vi "Handle Time Domain Data.vi"(8 "error in":errorcluster, 10 "Spkeaker On?":bool=TRUE, 11 "Cell Data in":refnum<class "PAS Cell Data.lvclass">) -> (0 "error out":errorcluster, 3 "Cell Data out":refnum<class "PAS Cell Data.lvclass">)   [LabVIEW 2014, in "PAS Library.lvlib" / "PAS Cell Data.lvclass"]
doc: "This VI handles the time domain data and any necessary transformation into the frequency domain. If the speaker is on, then the frequency domain data for the mic returned is the power spectrum (magnitude squared) and if the speaker is off, then the desired result is the magnitude. \n\nAlso, if the speaker is off, then the phase at the resonant frequency for the mic and photodiode are stored."
uses:
  PAS Cell Data.lvclass
  <vilib>/Analysis/4window.llb/windowTd.ctl
  PAS Cell Data.lvclass/PAS Cell Data.ctl
  <vilib>/measure/maspectr.llb/FFT Spectrum (Mag-Phase) for 1 Chan.vi
  <vilib>/Analysis/NI_AALPro.lvlib
  <vilib>/measure/NI_MAPro.lvlib
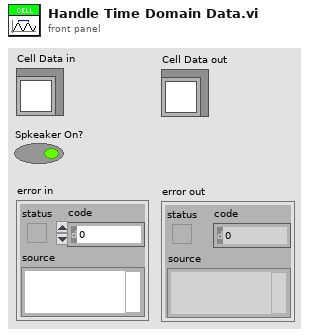
[diagram p1: front panel]
types:
  T1 = typedef "NI_AALPro.lvlib/windowTd.ctl" = u32
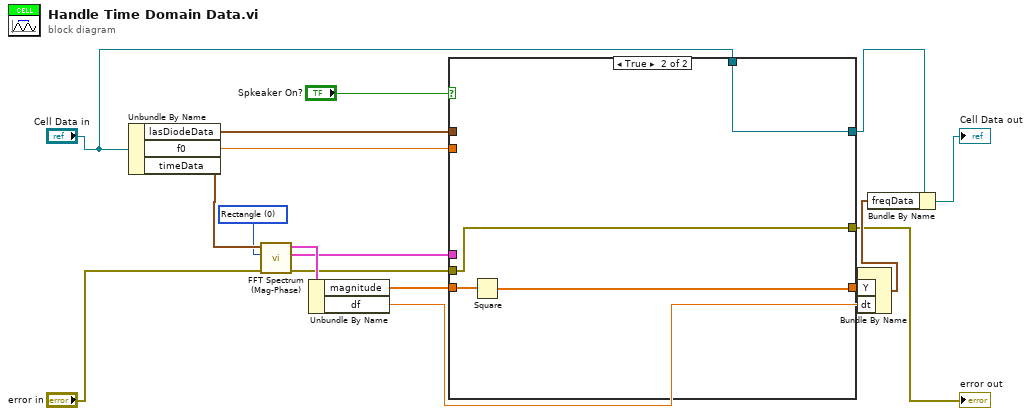
[diagram p0: block diagram]
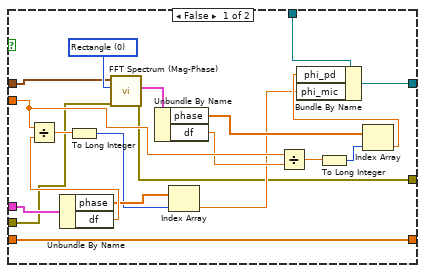
[diagram p2: hidden frame]
diagram:
  w14 = T1 0 items=["Rectangle"=0, "Hanning"=1, "Hamming"=2, "Blackman-Harris"=3, "Exact Blackman"=4, "Blackman"=5, "Flat Top"=6, "4 Term B-Harris "=7, "7 Term B-Harris"=8, "Low Sidelobe"=9, "Blackman Nuttall"=11, "Triangle"=30, "Bartlett-Hanning"=31, "Bohman"=32, "Parzen"=33, "Welch"=34, "Kaiser"=60, "Dolph-Chebyshev"=61, "Gaussian"=62] ("window")
  n1 = Unbundle By Name("Cell Data in") -> ("lasDiodeData"=w6:waveform(i16), "f0"=w7:sgl, "timeData"=w16:waveform(i16))
  n2 = call-poly <vilib>:"FFT Spectrum (Mag-Phase).vi"("error in (no error)"="error in", "window"=w14, "time signal"=w16) -> ("error out"=w2:errorcluster, "phase"=w8:cluster{"f0":dbl, "df":dbl, "phase":dbl[]}, "magnitude"=w17:cluster{"f0":dbl, "df":dbl, "magnitude":dbl[]})  [unwired: 4 in, 2 out]
  n3 = Unbundle By Name(w17) -> ("magnitude"=w12:dbl[], "df"=w5:dbl)
  n4 = case shown="True" "Spkeaker On?" {
    tunnel: w12 -> [w37 w41]
    tunnel: [w37 w40] -> w11
    tunnel: w8 -> [w33 _]
    tunnel: w7 -> [w28 _]
    tunnel: w6 -> [w35 _]
    tunnel: "Cell Data in" -> [w23 w39]
    tunnel: [w20 w39] -> w3
    tunnel: w2 -> [w19 w38]
    tunnel: [w18 w38] -> w1
    frame False {
      w36 = T1 0 items=["Rectangle"=0, "Hanning"=1, "Hamming"=2, "Blackman-Harris"=3, "Exact Blackman"=4, "Blackman"=5, "Flat Top"=6, "4 Term B-Harris "=7, "7 Term B-Harris"=8, "Low Sidelobe"=9, "Blackman Nuttall"=11, "Triangle"=30, "Bartlett-Hanning"=31, "Bohman"=32, "Parzen"=33, "Welch"=34, "Kaiser"=60, "Dolph-Chebyshev"=61, "Gaussian"=62] ("window")
      n5 = Unbundle By Name(w33) -> ("phase"=w31:dbl[], "df"=w32:dbl)
      n6 = Divide(x=w28, y=w32) -> (x/y=w34:dbl)
      n7 = To Long Integer(number=w34) -> (32bit integer=w30:i32)
      n8 = call-poly <vilib>:"FFT Spectrum (Mag-Phase).vi"("error in (no error)"=w19, "window"=w36, "time signal"=w35) -> ("error out"=w18:errorcluster, "phase"=w24:cluster{"f0":dbl, "df":dbl, "phase":dbl[]})  [unwired: 4 in, 3 out]
      n9 = Unbundle By Name(w24) -> ("phase"=w25:dbl[], "df"=w27:dbl)
      n10 = Index Array(array=w31, index=w30) -> (element=w21:dbl)
      n11 = Divide(x=w28, y=w27) -> (x/y=w29:dbl)
      n12 = To Long Integer(number=w29) -> (32bit integer=w26:i32)
      n13 = Index Array(array=w25, index=w26) -> (element=w22:dbl)
      n14 = Bundle By Name(cluster=w23, "phi_pd"=w22, "phi_mic"=w21) -> (w20:refnum<class "PAS Cell Data.lvclass">)
    }
    frame True {
      n15 = Square(x=w41) -> (x^2=w40:dbl[])
    }
  }
  "error out" <- w1
  n16 = Bundle By Name("Y"=w11, "dt"=w5) -> (w10:waveform(dbl))  [unwired: 1 out]
  n17 = Bundle By Name(cluster=w3, "freqData"=w10) -> (→"Cell Data out":refnum<class "PAS Cell Data.lvclass">)
